vi "Init.vi"(8 "error in (no error)":errorcluster, 9 "Channel Data (DBLs Only)":T1, 10 "Real-Time System Data":T2, 11 "Configuration Data":T3) -> (0 "error out":errorcluster, 1 "Channel Data (DBLs Only)":T1, 2 "Real-Time System Data":T2, 3 "Configuration Data":T3)   [LabVIEW 2014, in "RM interrupt timing Custom Device.lvlib"]
uses:
  RM interrupt timing Custom Device.lvlib
  Configuration Data.ctl
  Real-Time System Data.ctl
  Channel Data.ctl
  <instrlib>/GE 5565 PIORC/GE 5565 PIORC.lvlib
panel:
  # "Controls"
  # "Indicators"
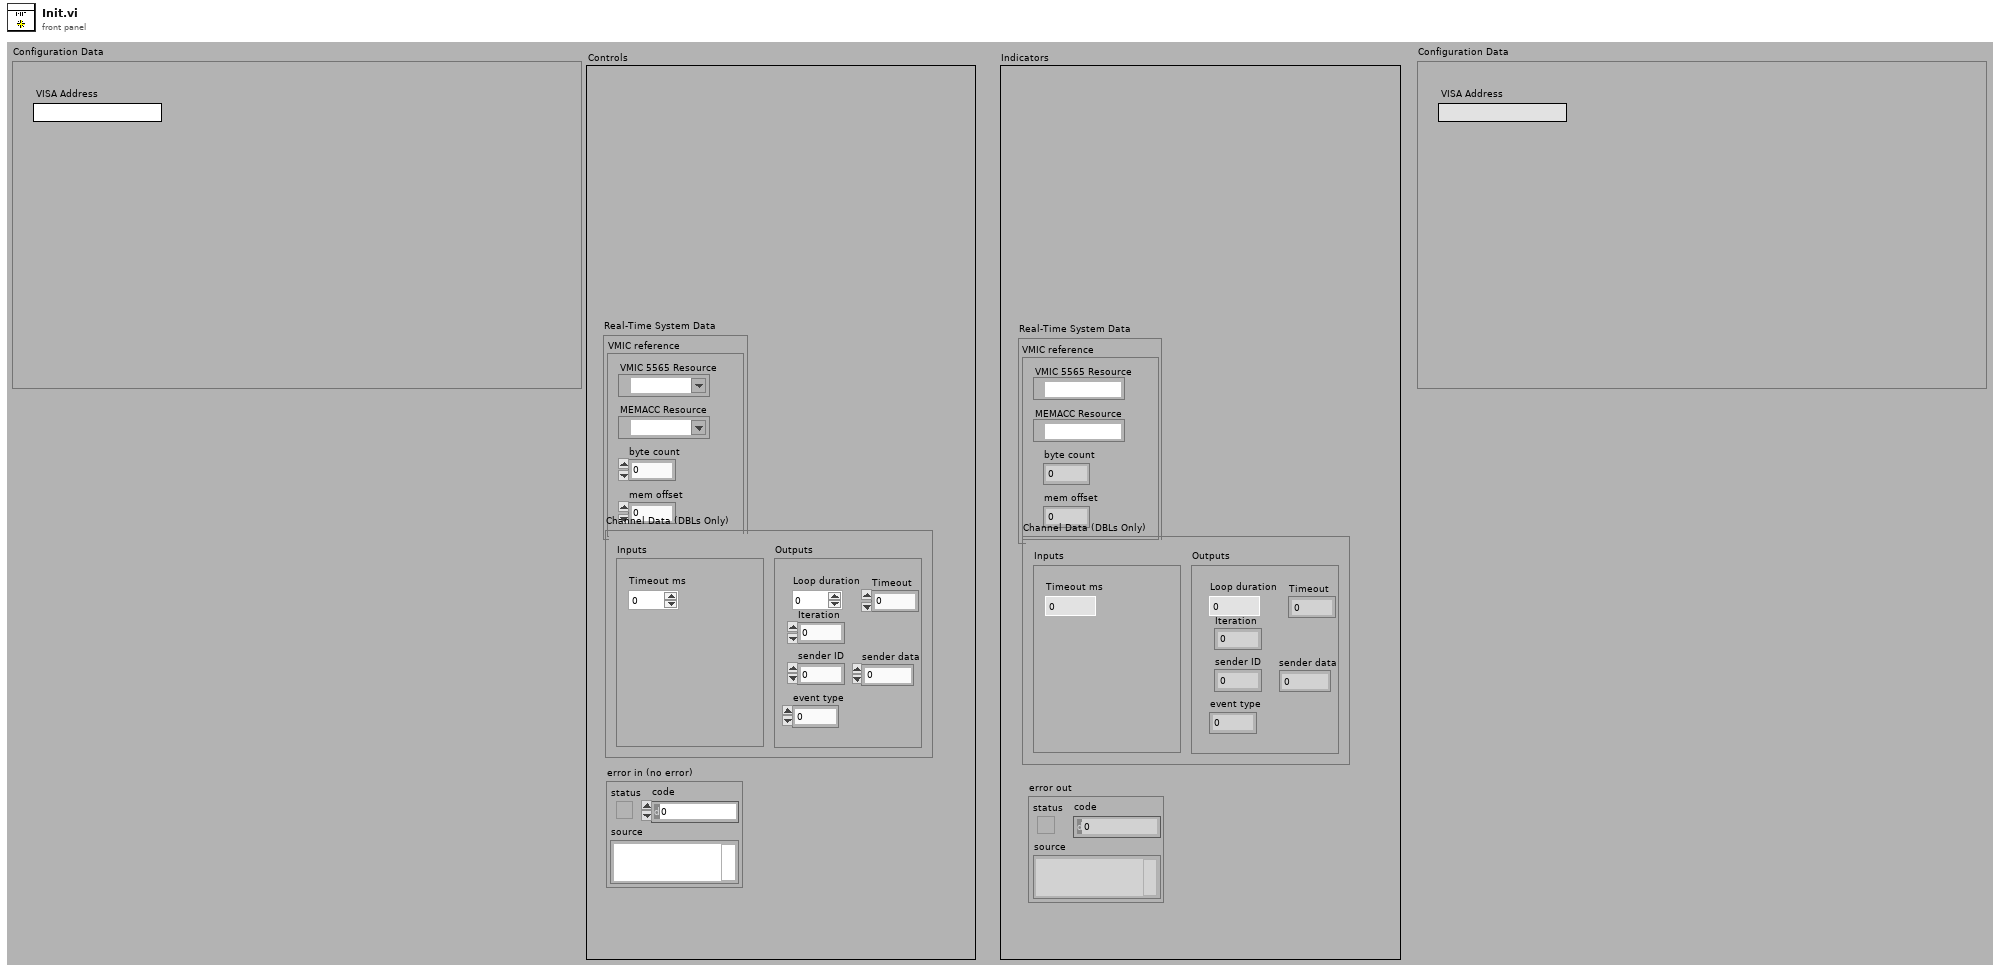
[diagram p1: front panel]
types:
  T1 = typedef "RM interrupt timing Custom Device.lvlib/Channel Data.ctl" = cluster{"Inputs":cluster{"Timeout ms":dbl}, "Outputs":cluster{"Loop duration":dbl, "Iteration":dbl, "Timeout":dbl, "sender data":dbl, "sender ID":dbl, "event type":dbl}}
  T2 = typedef "RM interrupt timing Custom Device.lvlib/Real-Time System Data.ctl" = cluster{"VMIC reference":cluster{"VMIC 5565 Resource":refnum<visa-resource-name>, "MEMACC Resource":refnum<visa-resource-name>, "byte count":u32, "mem offset":u32}}
  T3 = typedef "RM interrupt timing Custom Device.lvlib/Configuration Data.ctl" = cluster{"VISA Address":string}
  T4 = enum16{"link reset interrupt", "network interrupt 1", "network interrupt 2", "network interrupt 3", "network init interrupt", "all"}
  T5 = cluster{"VMIC 5565 Resource":refnum<visa-resource-name>, "MEMACC Resource":refnum<visa-resource-name>, "byte count":u32, "mem offset":u32}
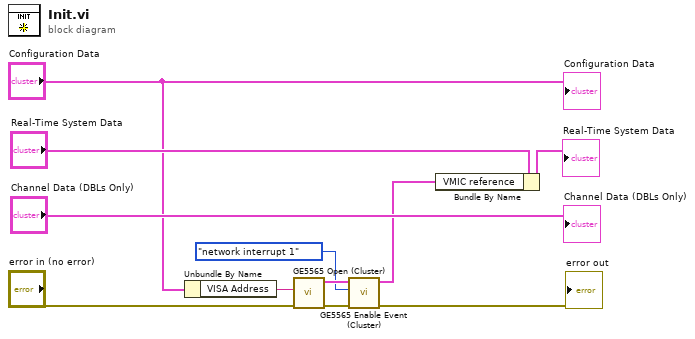
[diagram p0: block diagram]
diagram:
  n1 = Unbundle By Name("Configuration Data") -> ("VISA Address"=w3:string)
  n2 = call <instrlib>:"GE5565 Open (Cluster).vi"("error in (no error)"="error in (no error)", "VISA resource name (empty)"=w3) -> ("error out"=w8:errorcluster, "VMIC-5565"=w9:T5)  [unwired: 4 in]
  n3 = call <instrlib>:"GE5565 Enable Event (Cluster).vi"("error in (no error)"=w8, "event type (all)"=T4."network interrupt 1", "VMIC reference in"=w9) -> ("error out"=→"error out":errorcluster, "VMIC reference out"=w1:T5)  [unwired: 3 in]
  n4 = Bundle By Name(cluster="Real-Time System Data", "VMIC reference"=w1) -> (→"Real-Time System Data":T2)
  "Configuration Data" <- "Configuration Data"
  "Channel Data (DBLs Only)" <- "Channel Data (DBLs Only)"
